vi "Get Daemon Connections.vi"(8 "error in (no error)":errorcluster, 11 "Modbus slave in":refnum<class "Modbus Slave.lvclass">) -> (0 "error out":errorcluster, 2 "connections":T1[](array[typedef]), 3 "Modbus Slave out":refnum<class "Modbus Slave.lvclass">)   [LabVIEW 2015, in "Modbus Library.lvlib" / "Modbus Slave.lvclass"]
doc: "This VI is an accessor for the list of <B>connections</B> established to the Modbus slave instance. This accessor can be used as a property node."
uses:
  Modbus Slave.lvclass
  Network Protocol/Network Slave/TCP/Connection.ctl
  Modbus Slave.lvclass/Modbus Slave.ctl
  Network Protocol/Network Slave/TCP/TCP Slave.lvclass
  Network Protocol/Network Slave/TCP/TCP Slave.lvclass/TCP Slave.ctl
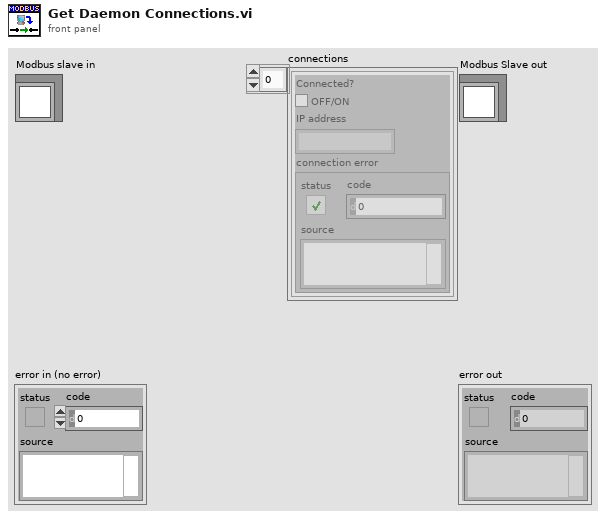
[diagram p1: front panel]
types:
  T1 = typedef "Modbus Library.lvlib/TCP Slave.lvclass/Connection.ctl" = cluster{"Connected?":bool, "IP address":string, "connection error":errorcluster}
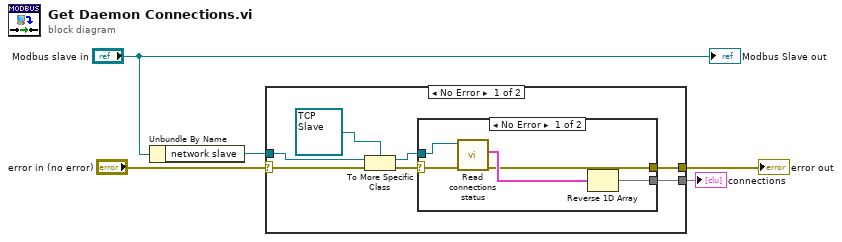
[diagram p0: block diagram]
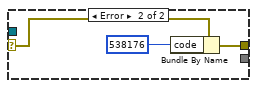
[diagram p2: hidden frame]
diagram:
  n1 = Unbundle By Name("Modbus slave in") -> ("network slave"=w4:refnum<class "Network Slave.lvclass">)
  n2 = case shown="No Error" "error in (no error)" {
    selector: "error in (no error)" -> [w10 w21]
    tunnel: w4 -> [w11 _]
    tunnel: [w7 _] -> w1
    tunnel: [w6 w21] -> w2
    frame No Error {
      n3 = To More Specific Class(target class=refnum<class "TCP Slave.lvclass"> refnum ("TCP Slave"), reference=w11, error in=w10) -> (specific class reference=w8:refnum<class "TCP Slave.lvclass">, error out=w9:errorcluster)
      n4 = case shown="No Error" w9 {
        selector: w9 -> [w15 w20]
        tunnel: w8 -> [w16 _]
        tunnel: [w17 _] -> w7
        tunnel: [w13 w19] -> w6
        frame No Error {
          n5 = call "Read connections status.vi"("error in (no error)"=w15, "TCP Slave in"=w16) -> ("error out"=w13:errorcluster, "Connections"=w14:T1[])  [unwired: 7 in, 1 out]
          n6 = Reverse 1D Array(array=w14) -> (reversed array=w17:T1[])
        }
        frame Error {
          n7 = Bundle By Name(cluster=w20, "code"=538176) -> (w19:errorcluster)
        }
      }
    }
    frame Error {
    }
  }
  "error out" <- w2
  "connections" <- w1
  "Modbus Slave out" <- "Modbus slave in"
